vi "Test Worker Handle Job.vi"(8 "error in (no error)":errorcluster, 11 "Worker Test in":refnum<class "Worker Test.lvclass">) -> (0 "error out":errorcluster, 3 "Worker Test out":refnum<class "Worker Test.lvclass">)   [LabVIEW 2020, in "Worker Test.lvclass"]
uses:
  Worker Test.lvclass
  Worker Test.lvclass/Worker Test.ctl
  <vilib>/Astemes/Triarc Framework/Process/Process.lvclass
  <vilib>/Astemes/Triarc Framework Test Suite/Mock Error Handler/Mock Error Handler.lvclass
  Processes/People/Workers/Worker/Worker.lvclass
  <vilib>/Astemes/LUnit/Test Case.lvclass
  C:/Git/astemes-triarc-examples/Coffee Shop/Processes/People/Person/Person.lvclass
  C:/Program Files (x86)/National Instruments/LabVIEW 2020/vi.lib/Astemes/Triarc Framework/View/View.lvclass
  C:/Program Files (x86)/National Instruments/LabVIEW 2020/vi.lib/Astemes/Triarc Framework/Process/Process.lvclass
  C:/Program Files (x86)/National Instruments/LabVIEW 2020/vi.lib/Astemes/Triarc Framework/Base/Base.lvclass
  C:/Program Files (x86)/National Instruments/LabVIEW 2020/vi.lib/Astemes/Triarc Framework/Error Handler Interface/Error Handler Interface.lvclass
  C:/Program Files (x86)/National Instruments/LabVIEW 2020/vi.lib/Astemes/Triarc Framework/Logging/Logging.lvclass
  C:/Git/astemes-triarc-examples/Coffee Shop/Processes/People/Workers/Worker/Worker.lvclass
  C:/Git/astemes-triarc-examples/Coffee Shop/Processes/People/Process Job/Job Handler.lvclass
  C:/Git/astemes-triarc-examples/Coffee Shop/Tests/Person Test/Person Test.lvclass
  C:/Program Files (x86)/National Instruments/LabVIEW 2020/vi.lib/Astemes/Triarc Framework Test Suite/View Test/View Test.lvclass
  C:/Program Files (x86)/National Instruments/LabVIEW 2020/vi.lib/Astemes/Triarc Framework Test Suite/Process Test/Process Test.lvclass
  C:/Program Files (x86)/National Instruments/LabVIEW 2020/vi.lib/Astemes/Triarc Framework Test Suite/Base Class Test/Base Test.lvclass
  C:/Program Files (x86)/National Instruments/LabVIEW 2020/vi.lib/Astemes/LUnit/Test Case.lvclass
  C:/Git/astemes-triarc-examples/Coffee Shop/Tests/Worker Test/Worker Test.lvclass
  C:/Program Files (x86)/National Instruments/LabVIEW 2020/vi.lib/Astemes/Triarc Framework Test Suite/Mock Error Handler/Mock Error Handler.lvclass
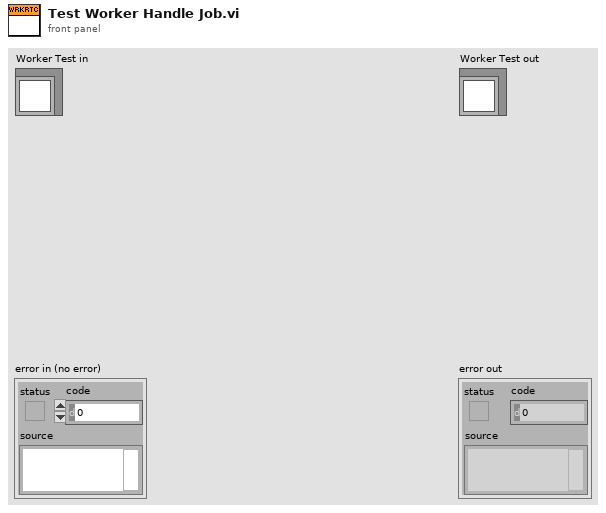
[diagram p1: front panel]
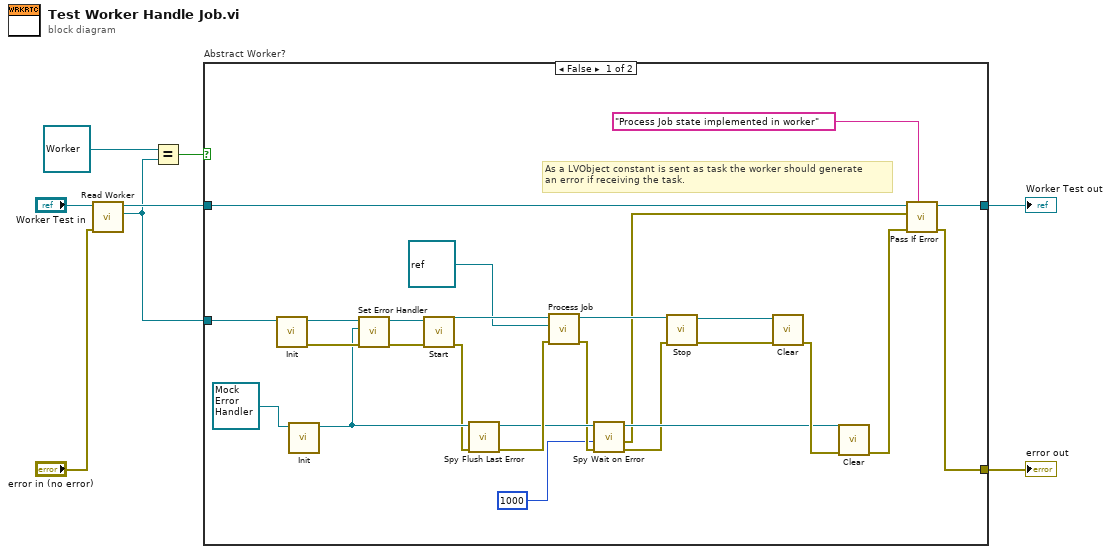
[diagram p0: block diagram]
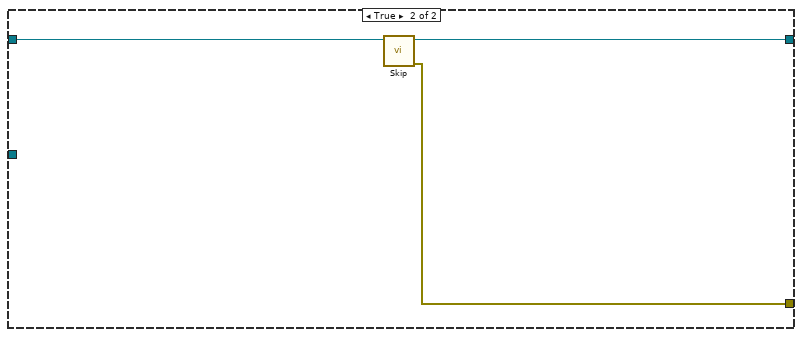
[diagram p2: hidden frame]
diagram:
  n1 = call "Read Worker.vi"("error in (no error)"="error in (no error)", "Worker Test in"="Worker Test in") -> ("Worker"=w2:refnum<class "Worker.lvclass">, "Worker Test out"=w5:refnum<class "Worker Test.lvclass">)  [unwired: 7 in, 1 out]
  n2 = Equal?(x=refnum<class "Worker.lvclass"> refnum ("Worker"), y=w2) -> (x = y?=w1:bool)
  n3 = case "Abstract Worker?" shown="False" w1 {
    tunnel: [w19 w35] -> w6
    tunnel: w5 -> [w18 w37]
    tunnel: [w17 w36] -> w4
    tunnel: w2 -> [w15 _]
    frame False {
      # "As a LVObject constant is sent as task the worker should generate \nan error if receiving the task."
      n4 = call-dynamic "Init.vi"("View In"=w15) -> ("error out"=w34:errorcluster, "View Out"=w30:refnum<class "Worker.lvclass">)  [unwired: 9 in]
      n5 = call-dynamic "Init.vi"("Mock Error Handler In"=refnum<class "Mock Error Handler.lvclass"> refnum) -> ("Mock Error Handler Out"=w27:refnum<class "Mock Error Handler.lvclass">)  [unwired: 9 in, 1 out]
      n6 = call <vilib>:"Set Error Handler.vi"("error in (no error)"=w34, "Error Handler"=w27, "Process In"=w30) -> ("error out"=w31:errorcluster, "Process Out"=w29:refnum<class "Worker.lvclass">)  [unwired: 7 in]
      n7 = call <vilib>:"Start.vi"("error in (no error)"=w31, "Process In"=w29) -> ("error out"=w26:errorcluster, "Process Out"=w25:refnum<class "Worker.lvclass">)  [unwired: 7 in, 1 out]
      n8 = call <vilib>:"Spy Flush Last Error.vi"("error in (no error)"=w26, "Mock Error Handler In"=w27) -> ("error out"=w24:errorcluster, "Mock Error Handler Out"=w14:refnum<class "Mock Error Handler.lvclass">)  [unwired: 7 in, 1 out]
      n9 = call-dynamic "Process Job.vi"("error in (no error)"=w24, "Job"=refnum<class> refnum ("Task"), "Worker In"=w25) -> ("error out"=w12:errorcluster, "Worker Out"=w22:refnum<class "Worker.lvclass">)  [unwired: 7 in]
      n10 = call <vilib>:"Spy Wait on Error.vi"("error in (no error)"=w12, "timeout in ms (-1)"=1000, "Mock Error Handler In"=w14) -> ("error out"=w9:errorcluster, "Errors"=w10:errorcluster, "Mock Error Handler Out"=w13:refnum<class "Mock Error Handler.lvclass">)  [unwired: 4 in, 2 out]
      n11 = call <vilib>:"Stop.vi"("error in (no error)"=w9, "Process In"=w22) -> ("error out"=w32:errorcluster, "Process Out"=w33:refnum<class "Worker.lvclass">)  [unwired: 7 in, 1 out]
      n12 = call-dynamic "Clear.vi"("error in (no error)"=w32, "View In"=w33) -> ("error out"=w21:errorcluster)  [unwired: 9 in]
      n13 = call-dynamic "Clear.vi"("error in (no error)"=w21, "Mock Process In"=w13) -> ("error out"=w20:errorcluster)  [unwired: 9 in]
      n14 = call <vilib>:"Pass If Error.vi"("Description"="Process Job state implemented in worker", "error in (no error)"=w20, "Assert error"=w10, "LUnit Test Case In"=w18) -> ("error out"=w19:errorcluster, "LUnit Test Case Out"=w17:refnum<class "Worker Test.lvclass">)  [unwired: 6 in]
    }
    frame True {
      n15 = call <vilib>:"Skip.vi"("LUnit Test Case In"=w37) -> ("error out"=w35:errorcluster, "LUnit Test Case Out"=w36:refnum<class "Worker Test.lvclass">)  [unwired: 9 in]
    }
  }
  "error out" <- w6
  "Worker Test out" <- w4
